vi "S2C_OM8257_Poly_LLT.vi"(8 "Error In":errorcluster, 10 "LLT":T1={"Leakage-Hi (V)"=6000.0, "Leakage-Lo (V)"=0.0, "Voltage-Hi (V)"=125.0, "Voltage-Lo (V)"=0.0, "Dwell (s)"=0.5, "Delay (s)"=1.0, "Offset (uA)"=10.0, "AC Src Voltage (V)"=115.0, "AC Src A-Hi (A)"=0.0, "AC Source"=FALSE, "AC Src Frequency"=60.0, "Auto Offset"=FALSE, "Reverse"=FALSE, "Active Link"=FALSE, "AC Src OC Fold"=FALSE, "Neutral"=FALSE, "Ground"=FALSE, "Leakage"=FALSE, "Ranging Mode"=FALSE, "AC Src Output"=TRUE, "AC Src Range"=TRUE, "Measure Device"=0, "Probe"=0, "Filter Mode"=0, "Scanner?"=FALSE, "Step Selection"=1, "Add Step"=FALSE, "Scan1"=1, "Scan2"=1, "Scan3"=1, "Scan4"=1, "Scan5"=1, "Scan6"=1, "Scan7"=1, "Scan8"=1, "Scan9"=1, "Scan10"=1, "Scan11"=1, "Scan12"=1, "Scan13"=1, "Scan14"=1, "Scan15"=1, "Scan16"=1} {"Scan16" min=0 max=2 step=1; "Scan15" min=0 max=2 step=1; "Scan14" min=0 max=2 step=1; "Scan13" min=0 max=2 step=1; "Scan12" min=0 max=2 step=1; "Scan11" min=0 max=2 step=1; "Scan10" min=0 max=2 step=1; "Scan9" min=0 max=2 step=1; "Scan8" min=0 max=2 step=1; "Scan7" min=0 max=2 step=1; "Scan6" min=0 max=2 step=1; "Scan5" min=0 max=2 step=1; "Scan4" min=0 max=2 step=1; "Scan3" min=0 max=2 step=1; "Scan2" min=0 max=2 step=1; "Scan1" min=0 max=2 step=1; "Measure Device" items=["UL544NP", "UL544P", "IEC60601 UL2601", "UL1563", "IEC60990 Fig4-U1 IEC60950", "IEC60990 Fig4-U2 IEC60950", "IEC60990 Fig5-U3", "External", "N/A", "Frequency Check"]; "Probe" items=["Ground To Line", "Probe-HI To Line", "Probe-HI To Probe-Lo"]; "Filter Mode" items=["AC+DC", "AC", "DC"]}, 11 "Settings":T2={"Driver"="Omnia8257", "Command"="CfgStep LLT", "Return"="ErrorStatus", "Parameters"="", "Timeout"=10.0}) -> (0 "Error Out":errorcluster, 3 "Response":string)   [LabVIEW 2015]
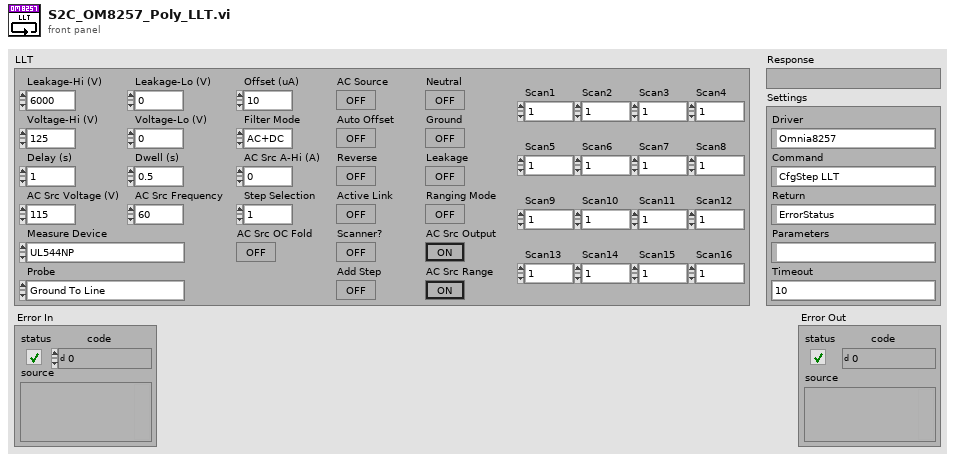
[diagram p1: front panel]
types:
  T1 = cluster{"Leakage-Hi (V)":dbl, "Leakage-Lo (V)":dbl, "Voltage-Hi (V)":dbl, "Voltage-Lo (V)":dbl, "Dwell (s)":dbl, "Delay (s)":dbl, "Offset (uA)":dbl, "AC Src Voltage (V)":dbl, "AC Src A-Hi (A)":dbl, "AC Source":bool, "AC Src Frequency":dbl, "Auto Offset":bool, "Reverse":bool, "Active Link":bool, "AC Src OC Fold":bool, "Neutral":bool, "Ground":bool, "Leakage":bool, "Ranging Mode":bool, "AC Src Output":bool, "AC Src Range":bool, "Measure Device":u16, "Probe":u16, "Filter Mode":u16, "Scanner?":bool, "Step Selection":i32, "Add Step":bool, "Scan1":i32, "Scan2":i32, "Scan3":i32, "Scan4":i32, "Scan5":i32, "Scan6":i32, "Scan7":i32, "Scan8":i32, "Scan9":i32, "Scan10":i32, "Scan11":i32, "Scan12":i32, "Scan13":i32, "Scan14":i32, "Scan15":i32, "Scan16":i32}
  T2 = cluster{"Driver":string, "Command":string, "Return":string, "Parameters":string, "Timeout":dbl}
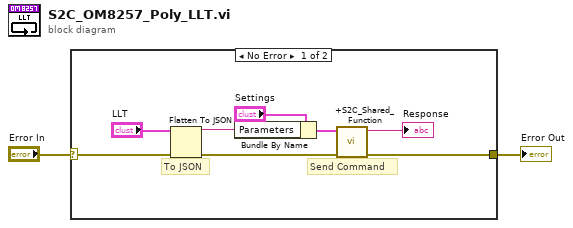
[diagram p0: block diagram]
diagram:
  n1 = case shown="No Error" "Error In" {
    selector: "Error In" -> [w6 w11]
    tunnel: [w5 w11] -> w1
    frame No Error {
      # "To JSON"
      # "Send Command"
      n2 = Flatten To JSON(anything="LLT", error in (no error)=w6) -> (JSON string=w7:string, 11:w9:errorcluster)  [unwired: 1 in]
      n3 = Bundle By Name(cluster="Settings", "Parameters"=w7) -> (w10:T2)
      n4 = call "+S2C_Shared_Function.vi"("Error In"=w9, "Settings"=w10) -> ("Error Out"=w5:errorcluster, "Response"=→"Response":string)  [unwired: 8 in]
    }
    frame Error {
    }
  }
  "Error Out" <- w1
